vi "Apply Firmware.vi"(8 "error in":errorcluster caption="error in (no error)", 11 "Target information":T3={"Hostname"="", "Serial number"="", "Product name"="", "Product code"=0, "System status"="", "Credential type"=enum."None/Unlocked", "User added?"=FALSE, "Primary NIC"={"MAC address"="", "IP Address Request Mode"=2, "IP address"="", "Subnet mask"="", "Gateway"="", "DNS server"=""}} {"Primary NIC"."IP Address Request Mode" items=["Static"=1, "DHCP/Link-Local"=2, "Link-Local Only"=4, "DHCP Only"=8]}) -> (0 "error out":errorcluster, 2 "Detailed Result":string, 3 "Firmware Status":T1=2 items=["update pending auto restart"=-4, "verifying new image"=-3, "writing/flashing new image"=-2, "waiting for image"=-1, "corrupt firmware, cannot run"=0, "no firmware installed"=1, ""=2, "update pending user restart"=3, "update pending user action"=4, "update attempt failed"=5])   [LabVIEW 2020]
doc: "This Vi will upgrade the RT device's firmware if it is not supported by SystemLink Client, which means firmware must be higher than version 6."
uses:
  Users/josferna/OneDrive - NI/Documents/Accounts&Proojects/Open Case Files/01072359 - Microsoft/rad-master/subVIs/Targets/TypeDefs/rad_Target Network Settings.ctl
  <vilib>/nisyscfg/Firmware Status.ctl
  <vilib>/nisyscfg/Upgrade Firmware (File).vi
  <vilib>/nisyscfg/Close (Hardware).vi
  <vilib>/nisyscfg/Close (System).vi
  <resource>/objmgr/nisysapi.rc
  <vilib>/nisyscfg/nisyscfg.lvlib
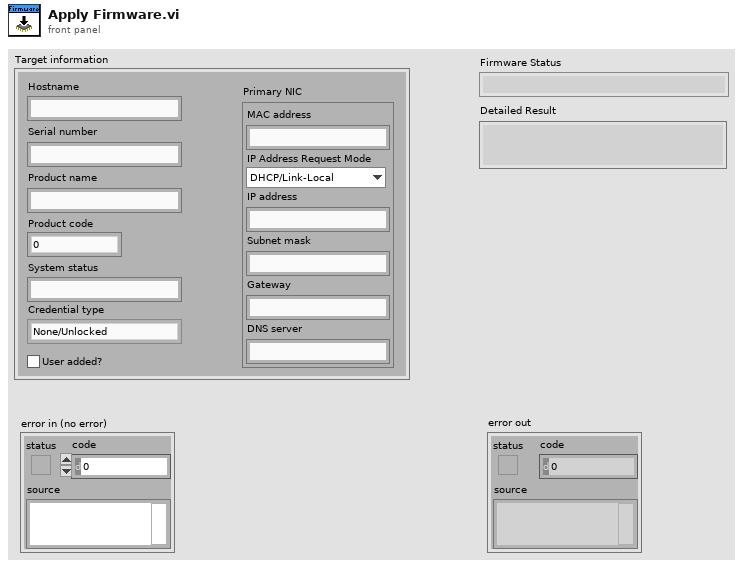
[diagram p1: front panel]
types:
  T1 = typedef "nisyscfg.lvlib/Firmware Status.ctl" = i32
  T2 = typedef "rad_Target Network Settings.ctl" = cluster{"MAC address":string, "IP Address Request Mode":i32, "IP address":string, "Subnet mask":string, "Gateway":string, "DNS server":string}
  T3 = cluster{"Hostname":string, "Serial number":string, "Product name":string, "Product code":i32, "System status":string, "Credential type":enum16{"None/Unlocked", "FTP Password", "NIAuth Credentials"}, "User added?":bool, "Primary NIC":T2}
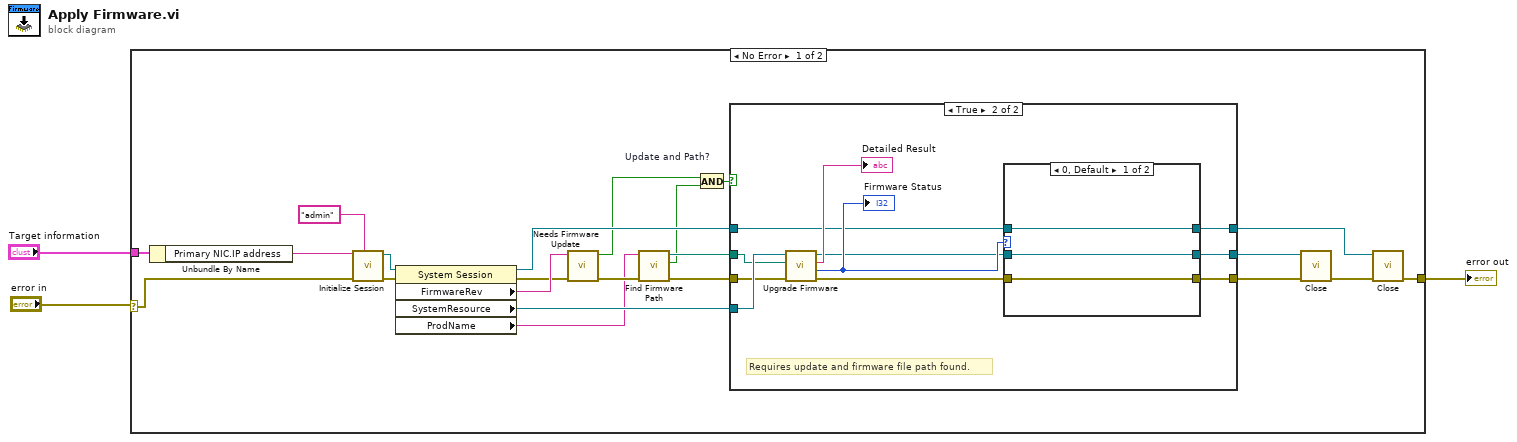
[diagram p0: block diagram]
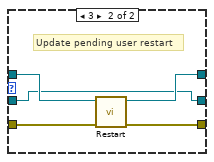
[diagram p3: hidden frame]
diagram:
  n1 = case shown="No Error" "error in" {
    selector: "error in" -> [w11 w48]
    tunnel: [w25 w48] -> w3
    tunnel: "Target information" -> [w18 _]
    frame No Error {
      n2 = Unbundle By Name(w18) -> ("Primary NIC.IP address"=w17:string)
      n3 = call <vilib>:"Initialize Session.vi"("User Name"="admin", "error in (no error)"=w11, "Target (localhost)"=w17) -> ("error out"=w21:errorcluster, "Session out"=w20:refnum<k21>)  [unwired: 7 in]
      n4 = property class="System Session"(reference=w20, error in=w21) -> (reference out=w14:refnum<k21>, error out=w15:errorcluster, "FirmwareRev"=w16:string, "SystemResource"=w19:refnum<k20>, "ProdName"=w8:string)
      n5 = call "Needs Firmware Update.vi"("error in (no error)"=w15, "FirmwareRev"=w16) -> ("error out"=w10:errorcluster, "Update?"=w5:bool)  [unwired: 8 in]
      n6 = call "Find Firmware Path.vi"("error in"=w10, "Product Name"=w8) -> ("error out"=w9:errorcluster, "Path Found?"=w4:bool, "Firmware Path"=w7:path)  [unwired: 7 in]
      n7 = And "Update and Path?"(x=w5, y=w4) -> (x .and. y?=w6:bool)
      n8 = case shown="True" w6 {
        tunnel: [w27 w30] -> w24
        tunnel: [w28 w33] -> w23
        tunnel: w19 -> [w27 w38]
        tunnel: w9 -> [w28 w37]
        tunnel: w14 -> [w26 w34]
        tunnel: [w26 w32] -> w12
        tunnel: w7 -> [_ w29]
        frame False {
          # "The system does not requires and update or the path was not found."
        }
        frame True {
          # "Requires update and firmware file path found."
          n9 = call-poly <vilib>:"Upgrade Firmware.vi"("error in (no error)"=w37, "Firmware File"=w29, "Resource in"=w38) -> ("error out"=w36:errorcluster, "Firmware Status"=w35:T1, "Detailed Result"=→"Detailed Result":string, "Resource out"=w31:refnum<k20>)  [unwired: 5 in]
          "Firmware Status" <- w35
          n10 = case shown="0, Default" w35 {
            tunnel: w36 -> [w41 w47]
            tunnel: w34 -> [w42 w46]
            tunnel: [w42 w45] -> w32
            tunnel: [w41 w44] -> w33
            tunnel: w31 -> [w40 w43]
            tunnel: [w40 w43] -> w30
            frame 0, Default {
            }
            frame 3 {
              # "Update pending user restart"
              n11 = call <vilib>:"Restart.vi"("error in (no error)"=w47, "Session in"=w46) -> ("error out"=w44:errorcluster, "Session out"=w45:refnum<k21>)  [unwired: 7 in, 1 out]
            }
          }
        }
      }
      n12 = call-poly <vilib>:"Close.vi"("error in (no error)"=w23, "Resource in"=w24) -> ("error out"=w13:errorcluster)  [unwired: 9 in]
      n13 = call-poly <vilib>:"Close.vi"("error in (no error)"=w13, "Session in"=w12) -> ("error out"=w25:errorcluster)  [unwired: 9 in]
    }
    frame Error {
    }
  }
  "error out" <- w3
